vi "Build Major Frame.vi"(8 "error in (no error)":errorcluster, 11 "Bus Controller XML Node":refnum<k20>) -> (0 "error out":errorcluster, 3 "Major Frame out":refnum<class "Major Frame.lvclass">)   [LabVIEW 2020]
doc: "Reads the Bus Controller node to produce an entire Major Frame schedule. The Major Frame, Minor Frames, and Messages all get constructed here."
uses:
  Frames & Messages/Major Frame/Major Frame.lvclass
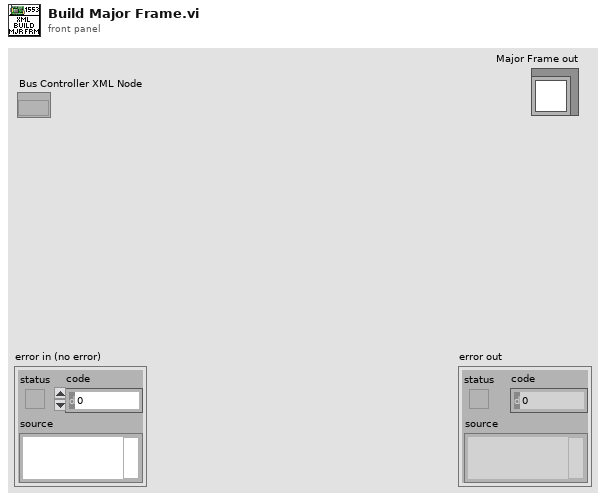
[diagram p1: front panel]
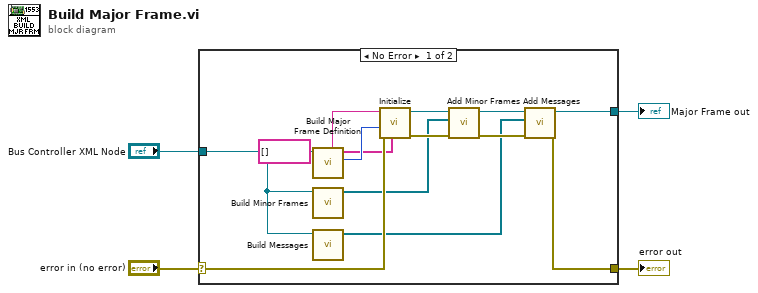
[diagram p0: block diagram]
diagram:
  n1 = case shown="No Error" "error in (no error)" {
    selector: "error in (no error)" -> [w10 w18]
    tunnel: [w9 w18] -> w3
    tunnel: "Bus Controller XML Node" -> [w8 _]
    tunnel: [w13 _] -> w1
    frame No Error {
      n2 = call "Build Major Frame Definition.vi"("Bus Controller XML Node"=w8) -> ("Minor Frame Rate"=w16:u16, "Major Frame ID"=w17:string)  [unwired: 7 in, 2 out]
      n3 = call "Build Minor Frames.vi"("Bus Controller XML Node"=w8) -> ("Minor Frames"=w7:refnum<class "Minor Frame.lvclass">[])  [unwired: 9 in, 1 out]
      n4 = call "Build Messages.vi"("Bus Controller XML Node"=w8) -> ("Messages"=w6:refnum<class "Message.lvclass">[])  [unwired: 9 in, 1 out]
      n5 = call "Initialize.vi"("Schedule"=string[] [], "error in (no error)"=w10, "Minor Frame Time (100 us)"=w16, "ID"=w17) -> ("error out"=w12:errorcluster, "Major Frame out"=w14:refnum<class "Major Frame.lvclass">)  [unwired: 6 in]
      n6 = call-dynamic "Add Minor Frames.vi"("error in (no error)"=w12, "Minor Frames"=w7, "Major Frame in"=w14) -> ("error out"=w11:errorcluster, "Major Frame out"=w15:refnum<class "Major Frame.lvclass">)  [unwired: 7 in]
      n7 = call-dynamic "Add Messages.vi"("error in (no error)"=w11, "Messages"=w6, "Major Frame in"=w15) -> ("error out"=w9:errorcluster, "Major Frame out"=w13:refnum<class "Major Frame.lvclass">)  [unwired: 7 in]
    }
    frame Error {
    }
  }
  "error out" <- w3
  "Major Frame out" <- w1
